vi "NATIVE_DATA_FORMAT_COUNT.vi"() -> (3 "NATIVE_DATA_FORMAT_COUNT":i32=64)   [LabVIEW 2020, in "G-Audio.lvlib"]
uses:
  G-Audio.lvlib
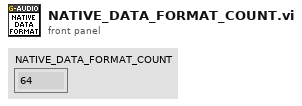
[diagram p1: front panel]
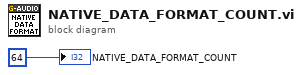
[diagram p0: block diagram]
diagram:
  "NATIVE_DATA_FORMAT_COUNT" <- 64
